vi "operaciones matematicas.vi"() -> ()   [LabVIEW 2011]
panel:
  out "Multiplicar":dbl
  out "Division":dbl
  out "Resta":dbl
  out "Suma":dbl
  in  "Numero2":dbl
  in  "Numero 1":dbl
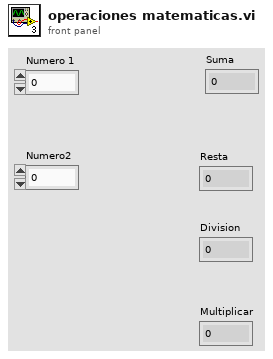
[diagram p1: front panel]
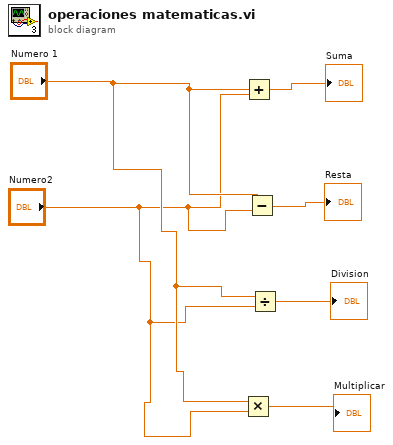
[diagram p0: block diagram]
diagram:
  n1 = Multiply(x="Numero 1", y="Numero2") -> (x*y=→"Multiplicar":dbl)
  n2 = Add(x="Numero 1", y="Numero2") -> (x+y=→"Suma":dbl)
  n3 = Subtract(x="Numero 1", y="Numero2") -> (x-y=→"Resta":dbl)
  n4 = Divide(x="Numero 1", y="Numero2") -> (x/y=→"Division":dbl)
